vi "load_class-multiple.vi"(8 "error in (no error)":errorcluster, 11 "class_folder":path) -> (0 "error out":errorcluster, 3 "lv_post_installer []":refnum<class "lv-post-installer.lvclass">[](array[class]))   [LabVIEW 2015, in "lv-post-installer.lvlib"]
uses:
  lv-post-installer.lvlib
  classes/lv-post-installer/lv-post-installer.lvclass
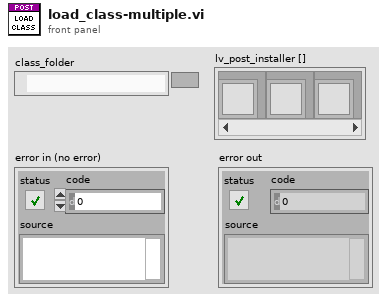
[diagram p1: front panel]
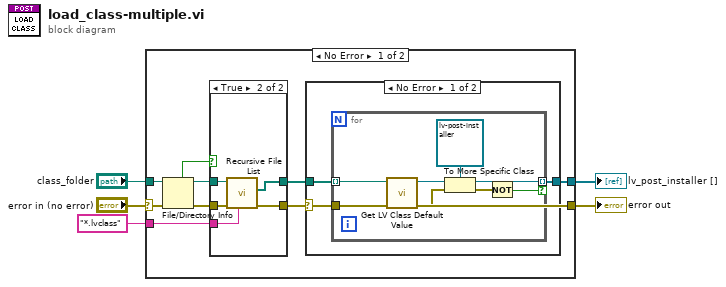
[diagram p0: block diagram]
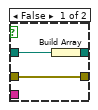
[diagram p2: hidden frame]
diagram:
  n1 = case shown="No Error" "error in (no error)" {
    selector: "error in (no error)" -> [w12 w34]
    tunnel: [w14 _] -> w5
    tunnel: [w7 w34] -> w4
    tunnel: "class_folder" -> [w13 _]
    tunnel: "*.lvclass" -> [w6 _]
    frame No Error {
      n2 = File/Directory Info(path=w13, error in=w12) -> (path out=w11:path, directory=w9:bool, error out=w10:errorcluster)  [unwired: 4 out]
      n3 = case shown="True" w9 {
        tunnel: w11 -> [w17 w21]
        tunnel: w10 -> [w15 w22]
        tunnel: [w15 w20] -> w7
        tunnel: [w16 w19] -> w8
        tunnel: w6 -> [_ w18]
        frame False {
          n4 = Build Array(w17) -> (w16:path[])
        }
        frame True {
          n5 = call <vilib>:"Recursive File List.vi"("pattern"=w18, "error in (no error)"=w22, "Folder Path"=w21) -> ("error out"=w20:errorcluster, "All Files in Dir"=w19:path[])  [unwired: 4 in, 3 out]
        }
      }
      n6 = case shown="No Error" w7 {
        selector: w7 -> [w23 _]
        tunnel: [w25 _] -> w14
        tunnel: w8 -> [w24 _]
        frame No Error {
          n7 = for {
            tunnel: [w31] -> w25 mode=indexing if=w27
            tunnel: w24 -> [w29] mode=indexing
            tunnel: w23 -> [w28]
            n8 = call <vilib>:"Get LV Class Default Value.vi"("error in (no error)"=w28, "class path"=w29) -> ("error out"=w32:errorcluster, "object"=w33:refnum<class>)  [unwired: 8 in]
            n9 = To More Specific Class(target class=refnum<class "lv-post-installer.lvclass"> refnum ("lv-post-installer.lvlib:lv-post-installer.lvclass"), reference=w33, error in=w32) -> (specific class reference=w31:refnum<class "lv-post-installer.lvclass">, error out=w26:errorcluster)
            n10 = Not(x=w26) -> (.not. x?=w27:bool)
          }
        }
        frame Error {
        }
      }
    }
    frame Error {
    }
  }
  "error out" <- w4
  "lv_post_installer []" <- w5
